vi "Run_Core.vi"(0 "Message Popup in":refnum<class "Timing Functions.lvclass">, 11 "error in (no error)":errorcluster) -> (4 "Message Popup out":refnum<class "Timing Functions.lvclass">, 6 "Return":variant, 15 "error out":errorcluster)   [LabVIEW 2019, in "Timing Functions.lvclass"]
uses:
  Timing Functions.lvclass
  Timing Functions.lvclass/Timing Functions.ctl
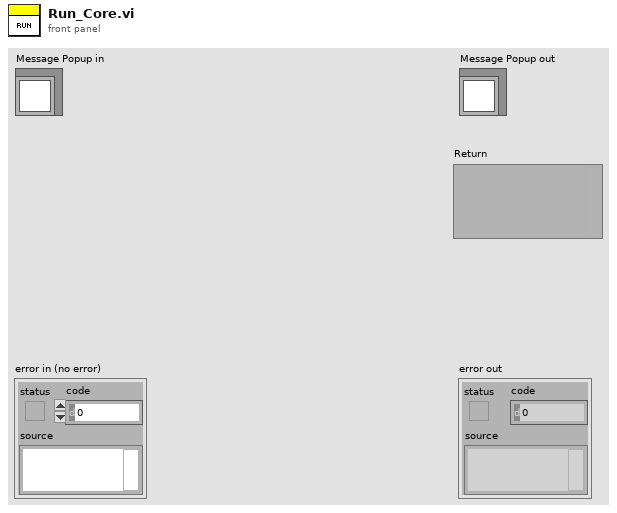
[diagram p1: front panel]
types:
  T1 = typedef "Timing Functions.lvclass/Function List.ctl" = enum16{"High Res Time", "Wait", "Get Date and Time"}
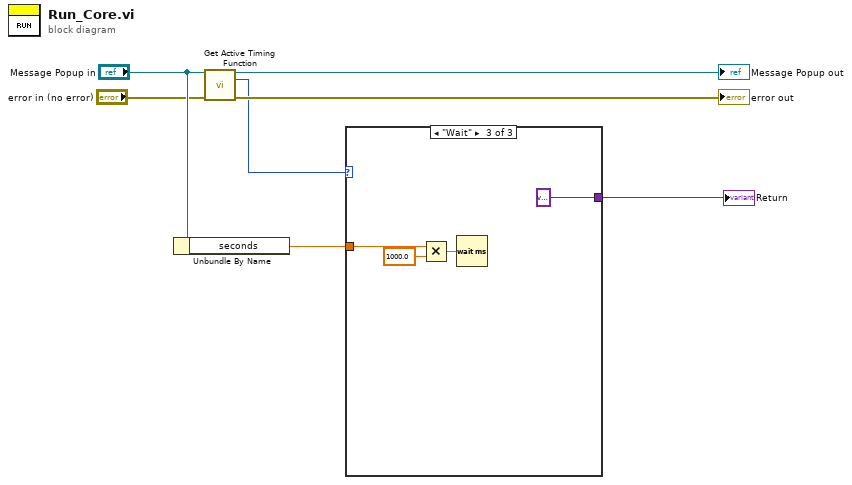
[diagram p0: block diagram]
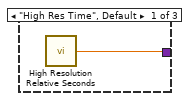
[diagram p2: hidden frame]
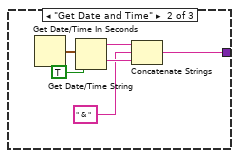
[diagram p3: hidden frame]
diagram:
  n1 = Unbundle By Name("Message Popup in") -> ("seconds"=w7:dbl)
  n2 = call "Get Active Timing Function.vi"("Timing Functions in"="Message Popup in", "error in (no error)"="error in (no error)") -> ("Timing Functions out"=→"Message Popup out":refnum<class "Timing Functions.lvclass">, "Function List"=w2:T1, "error out"=→"error out":errorcluster)  [unwired: 11 in]
  n3 = case shown="\"Wait\"" w2 {
    tunnel: w7 -> [_ _ w18]
    tunnel: [w8 w9 variant] -> w1
    frame "High Res Time", Default {
      n4 = call <vilib>:"High Resolution Relative Seconds.vi"() -> ("relative seconds"=w8:dbl)
    }
    frame "Get Date and Time" {
      n5 = Get Date/Time In Seconds() -> (seconds since 1Jan1904=w14:timestamp)
      n6 = Get Date/Time String(seconds (now)=w14, want seconds? (F)=TRUE) -> (date string=w13:string, time string=w12:string)  [unwired: 1 in]
      n7 = Concatenate Strings(w13, " & " ("string"), w12) -> (w9:string)
    }
    frame "Wait" {
      n8 = Multiply(x=w18, y=1000.0) -> (x*y=w16:dbl)
      n9 = Wait (ms)(milliseconds to wait=w16) -> ()  [unwired: 1 out]
    }
  }
  "Return" <- w1
